vi "Reconcile Attributes for Prefix.vi"(7 "Prefix":T1, 9 "Secure In":bool, 10 "Path In":string, 11 "Domain In":string) -> (1 "Secure":string, 2 "Path":string, 3 "Domain":string)   [LabVIEW 2020, in "HTTP Utils.lvlib" / "Cookie.lvclass"]
uses:
  Cookie.lvclass
  Cookie Prefix.ctl
  HTTP Utils.lvlib
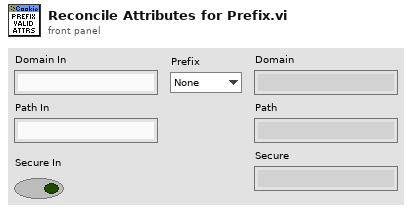
[diagram p1: front panel]
types:
  T1 = typedef "HTTP Utils.lvlib/Cookie Prefix.ctl" = enum16{"None", "Host", "Secure"}
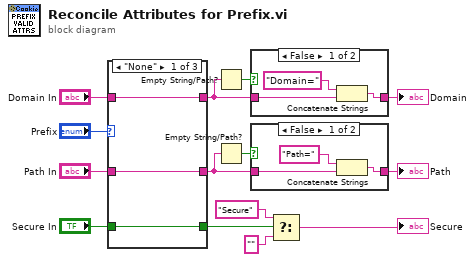
[diagram p0: block diagram]
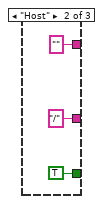
[diagram p2: hidden frame]
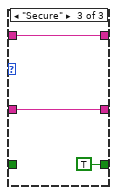
[diagram p3: hidden frame]
diagram:
  n1 = case shown="\"None\"" "Prefix" {
    tunnel: "Secure In" -> [w15 _ _]
    tunnel: "Path In" -> [w16 _ w21]
    tunnel: "Domain In" -> [w17 _ w22]
    tunnel: [w17 "" ("Domain In") w22] -> w9
    tunnel: [w16 "/" ("Path In") w21] -> w5
    tunnel: [w15 TRUE ("Secure In") TRUE ("Secure In")] -> w4
    frame "None" {
    }
    frame "Host" {
    }
    frame "Secure" {
    }
  }
  n2 = Empty String/Path?(string/path=w9) -> (empty?=w10:bool)
  n3 = Empty String/Path?(string/path=w5) -> (empty?=w7:bool)
  n4 = case shown="False" w10 {
    tunnel: w9 -> [w26 w27]
    tunnel: [w25 w27] -> w8
    frame False {
      n5 = Concatenate Strings("Domain=", w26) -> (w25:string)
    }
    frame True {
    }
  }
  "Domain" <- w8
  n6 = case shown="False" w7 {
    tunnel: w5 -> [w30 w31]
    tunnel: [w29 w31] -> w6
    frame False {
      n7 = Concatenate Strings("Path=", w30) -> (w29:string)
    }
    frame True {
    }
  }
  "Path" <- w6
  n8 = Select(t="Secure", s=w4, f="") -> (s? t:f=→"Secure":string)
